vi "Init Shared and Network Variables.vi"(8 "error in (no error)":errorcluster) -> (0 "error out":errorcluster)   [LabVIEW 2024]
uses:
  Type Definitions/FIFO_Health.ctl
  Type Definitions/DIO_Cluster.ctl
  Type Definitions/FPGA_routine_pulsing_typedef.ctl
  Type Definitions/CPU_and_memory.ctl
panel:
  out "current time":timestamp
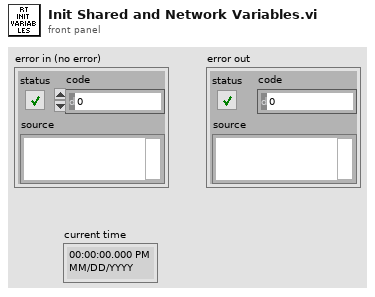
[diagram p1: front panel]
types:
  T1 = typedef "CPU_and_memory.ctl" = cluster{"CPU 1 (%)":dbl, "CPU 2 (%)":dbl, "Free Virtual\nMemory(%)":dbl, "Free Hard drive space (%)":dbl, "Free Physical\n Memory (%)":dbl}
  T2 = typedef "FPGA_routine_pulsing_typedef.ctl" = cluster{"Pulsing":bool, "Pulse duration (uS)":u32, "Pulse Period (uS)":u32}
  T3 = typedef "DIO_Cluster.ctl" = cluster{"DIO0":bool, "DIO1":bool, "DIO2":bool, "DIO3":bool}
  T4 = typedef "FIFO_Health.ctl" = cluster{"Elements in RT FIFO":i32, "Network Stream Full":bool, "RT FIFO Full":bool, "FPGA AI Underflow":bool, "FPGA FIFO Full":bool, "FPGA Loop Timing Off":bool, "timestamp":timestamp, "Stream Size":u32, "Packet Size":u32}
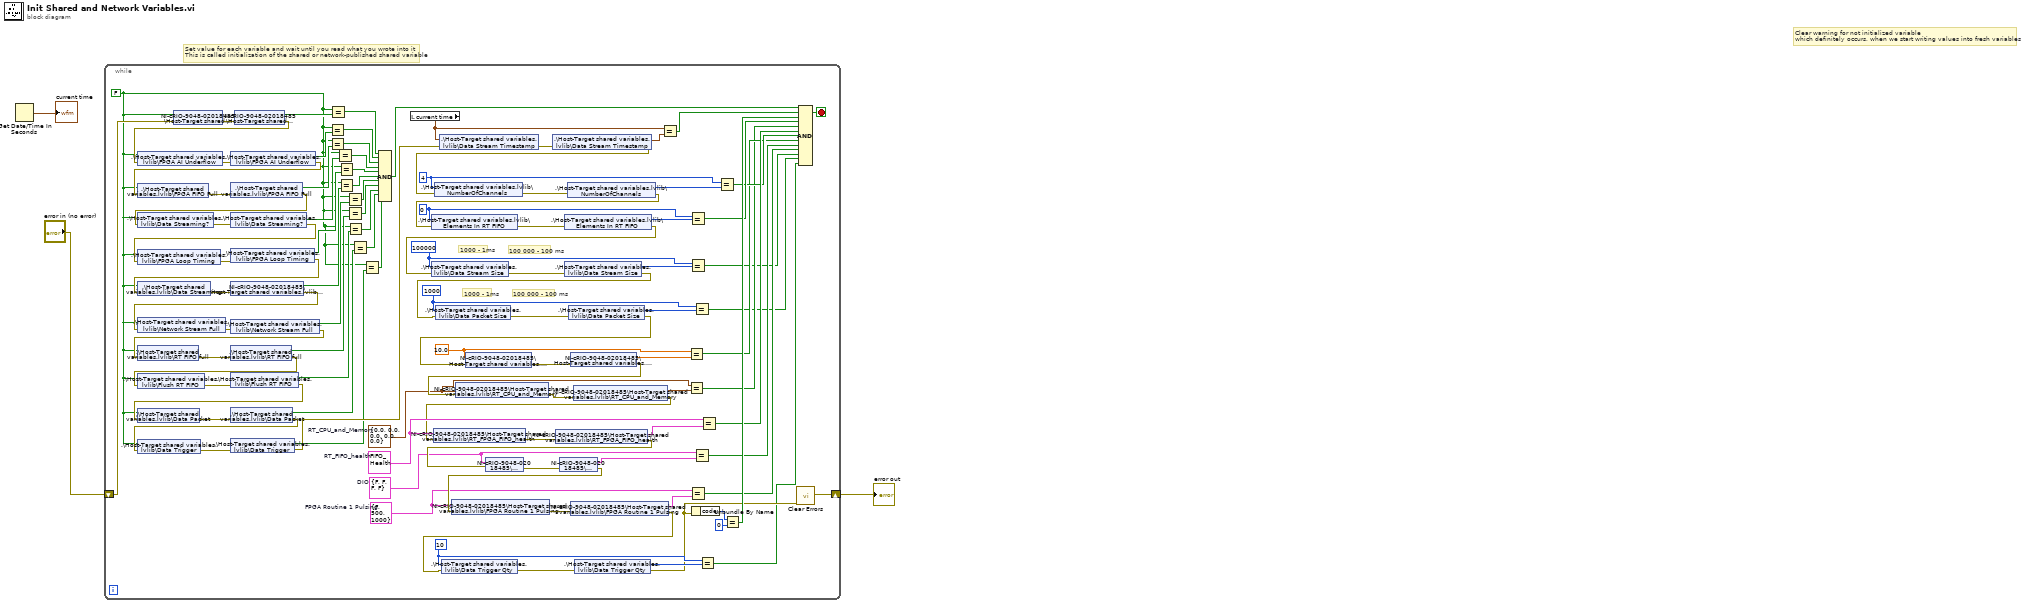
[diagram p0: block diagram]
diagram:
  # "Set value for each variable and wait until you read what you wrote into it\nThis is called initialization of the shared or network-published shared variable"
  # "Clear warning for not initialized variable\nwhich definitely occurs, when we start writing values into fresh variables"
  n1 = Get Date/Time In Seconds() -> (seconds since 1Jan1904=→"current time":timestamp)
  n2 = while {
    shift-right: [w101] -> w2
    shift-left: "error in (no error)" -> [w100]
    stop <- w94 stop-if-true
    w7 = u32 10 ("Elements In RT FIFO AI")
    w19 = u32 1000 ("Elements In RT FIFO AI")
    w24 = u32 100000 ("Elements In RT FIFO AI")
    w45 = T1 {"CPU 1 (%)"=0.0, "CPU 2 (%)"=0.0, "Free Virtual\nMemory(%)"=0.0, "Free Hard drive space (%)"=0.0, "Free Physical\n Memory (%)"=0.0}  # RT_CPU_and_Memory
    w52 = T2 {"Pulsing"=FALSE, "Pulse duration (uS)"=500, "Pulse Period (uS)"=1000}  # FPGA Routine 1 Pulsing
    w56 = T3 {"DIO0"=FALSE, "DIO1"=FALSE, "DIO2"=FALSE, "DIO3"=FALSE}  # DIO
    w61 = 10.0 ("Binning Time")
    w75 = u8 4 ("NumberOfChannels")
    w81 = T4 {"Elements in RT FIFO"=0, "Network Stream Full"=FALSE, "RT FIFO Full"=FALSE, "FPGA AI Underflow"=FALSE, "FPGA FIFO Full"=FALSE, "FPGA Loop Timing Off"=FALSE, "timestamp"=timestamp(0 s since 1904-01-01), "Stream Size"=0, "Packet Size"=0}  # RT_FIFO_health
    w27 = 0 ("Elements In RT FIFO AI")
    w12 = FALSE
    # "100 000 - 100 ms"
    # "1000 - 1ms"
    # "100 000 - 100 ms"
    # "1000 - 1ms"
    n3 = shared-variable "NI-cRIO-9048-02018485\\Host-Target shared variables.lvlib\\Stop RT"(w12, error in=w100) -> (error out=w109:errorcluster)
    n4 = shared-variable "NI-cRIO-9048-02018485\\Host-Target shared variables.lvlib\\Stop RT"(error in=w109) -> (w108:bool, error out=w67:errorcluster)
    n5 = shared-variable ".\\Host-Target shared variables.lvlib\\FPGA AI Underflow"(w12, error in=w67) -> (error out=w43:errorcluster)
    n6 = shared-variable ".\\Host-Target shared variables.lvlib\\FPGA AI Underflow"(error in=w43) -> (w36:bool, error out=w66:errorcluster)
    n7 = shared-variable ".\\Host-Target shared variables.lvlib\\FPGA FIFO Full"(w12, error in=w66) -> (error out=w69:errorcluster)
    n8 = shared-variable ".\\Host-Target shared variables.lvlib\\FPGA FIFO Full"(error in=w69) -> (w35:bool, error out=w68:errorcluster)
    n9 = shared-variable ".\\Host-Target shared variables.lvlib\\Data Streaming?"(w12, error in=w68) -> (error out=w107:errorcluster)
    n10 = shared-variable ".\\Host-Target shared variables.lvlib\\Data Streaming?"(error in=w107) -> (w34:bool, error out=w72:errorcluster)
    n11 = shared-variable ".\\Host-Target shared variables.lvlib\\FPGA Loop Timing"(w12, error in=w72) -> (error out=w73:errorcluster)
    n12 = shared-variable ".\\Host-Target shared variables.lvlib\\FPGA Loop Timing"(error in=w73) -> (w33:bool, error out=w71:errorcluster)
    n13 = shared-variable ".\\Host-Target shared variables.lvlib\\Data Streaming"(w12, error in=w71) -> (error out=w110:errorcluster)
    n14 = shared-variable "NI-cRIO-9048-02018485\\Host-Target shared variables.lvlib\\Data Streaming"(error in=w110) -> (w32:bool, error out=w90:errorcluster)
    n15 = shared-variable ".\\Host-Target shared variables.lvlib\\Network Stream Full"(w12, error in=w90) -> (error out=w92:errorcluster)
    n16 = shared-variable ".\\Host-Target shared variables.lvlib\\Network Stream Full"(error in=w92) -> (w31:bool, error out=w89:errorcluster)
    n17 = shared-variable ".\\Host-Target shared variables.lvlib\\RT FIFO full"(w12, error in=w89) -> (error out=w91:errorcluster)
    n18 = shared-variable ".\\Host-Target shared variables.lvlib\\RT FIFO full"(error in=w91) -> (w30:bool, error out=w41:errorcluster)
    n19 = shared-variable ".\\Host-Target shared variables.lvlib\\Flush RT FIFO"(w12, error in=w41) -> (error out=w42:errorcluster)
    n20 = shared-variable ".\\Host-Target shared variables.lvlib\\Flush RT FIFO"(error in=w42) -> (w40:bool, error out=w37:errorcluster)
    n21 = shared-variable ".\\Host-Target shared variables.lvlib\\Data Packet"(w12, error in=w37) -> (error out=w38:errorcluster)
    n22 = shared-variable ".\\Host-Target shared variables.lvlib\\Data Packet"(error in=w38) -> (w29:bool, error out=w14:errorcluster)
    n23 = shared-variable ".\\Host-Target shared variables.lvlib\\Data Trigger"(w12, error in=w14) -> (error out=w15:errorcluster)
    n24 = shared-variable ".\\Host-Target shared variables.lvlib\\Data Trigger"(error in=w15) -> (w11:bool, error out=w13:errorcluster)
    n25 = Equal?(x=w12, y=w36) -> (x = y?=w105:bool)
    n26 = Equal?(x=w12, y=w35) -> (x = y?=w104:bool)
    n27 = Equal?(x=w12, y=w108) -> (x = y?=w106:bool)
    n28 = Equal?(x=w12, y=w34) -> (x = y?=w88:bool)
    n29 = Equal?(x=w12, y=w33) -> (x = y?=w87:bool)
    n30 = Equal?(x=w12, y=w32) -> (x = y?=w70:bool)
    n31 = Equal?(x=w12, y=w31) -> (x = y?=w64:bool)
    n32 = Equal?(x=w12, y=w30) -> (x = y?=w65:bool)
    n33 = Equal?(x=w12, y=w40) -> (x = y?=w39:bool)
    n34 = Equal?(x=w12, y=w29) -> (x = y?=w28:bool)
    n35 = Equal?(x=w12, y=w11) -> (x = y?=w10:bool)
    n36 = Compound Arithmetic op=AND(w106, w105, w104, w88, w87, w70, w64, w65, w39, w28, w10) -> (w97:bool)
    n37 = local read "current time"() -> (w93:timestamp)
    n38 = shared-variable ".\\Host-Target shared variables.lvlib\\Data Stream Timestamp"(w93, error in=w13) -> (error out=w99:errorcluster)
    n39 = shared-variable ".\\Host-Target shared variables.lvlib\\Data Stream Timestamp"(error in=w99) -> (w98:timestamp, error out=w79:errorcluster)
    n40 = shared-variable ".\\Host-Target shared variables.lvlib\\NumberOfChannels"(w75, error in=w79) -> (error out=w78:errorcluster)
    n41 = shared-variable ".\\Host-Target shared variables.lvlib\\NumberOfChannels"(error in=w78) -> (w76:u8, error out=w77:errorcluster)
    n42 = shared-variable ".\\Host-Target shared variables.lvlib\\Elements In RT FIFO"(w27, error in=w77) -> (error out=w86:errorcluster)
    n43 = shared-variable ".\\Host-Target shared variables.lvlib\\Elements In RT FIFO"(error in=w86) -> (w85:i32, error out=w23:errorcluster)
    n44 = shared-variable ".\\Host-Target shared variables.lvlib\\Data Stream Size"(w24, error in=w23) -> (error out=w26:errorcluster)
    n45 = shared-variable ".\\Host-Target shared variables.lvlib\\Data Stream Size"(error in=w26) -> (w25:u32, error out=w18:errorcluster)
    n46 = shared-variable ".\\Host-Target shared variables.lvlib\\Data Packet Size"(w19, error in=w18) -> (error out=w21:errorcluster)
    n47 = shared-variable ".\\Host-Target shared variables.lvlib\\Data Packet Size"(error in=w21) -> (w20:u32, error out=w17:errorcluster)
    n48 = shared-variable "NI-cRIO-9048-02018485\\Host-Target shared variables.lvlib\\Binning Time"(w61, error in=w17) -> (error out=w63:errorcluster)
    n49 = shared-variable "NI-cRIO-9048-02018485\\Host-Target shared variables.lvlib\\Binning Time"(error in=w63) -> (w62:dbl, error out=w48:errorcluster)
    n50 = shared-variable "NI-cRIO-9048-02018485\\Host-Target shared variables.lvlib\\RT_CPU_and_Memory"(w45, error in=w48) -> (error out=w49:errorcluster)
    n51 = shared-variable "NI-cRIO-9048-02018485\\Host-Target shared variables.lvlib\\RT_CPU_and_Memory"(error in=w49) -> (w46:T1, error out=w47:errorcluster)
    n52 = shared-variable "NI-cRIO-9048-02018485\\Host-Target shared variables.lvlib\\RT_FPGA_FIFO_health"(w81, error in=w47) -> (error out=w83:errorcluster)
    n53 = shared-variable "NI-cRIO-9048-02018485\\Host-Target shared variables.lvlib\\RT_FPGA_FIFO_health"(error in=w83) -> (w82:T4, error out=w59:errorcluster)
    n54 = shared-variable "NI-cRIO-9048-02018485\\Host-Target shared variables.lvlib\\DIO"(w56, error in=w59) -> (error out=w58:errorcluster)
    n55 = shared-variable "NI-cRIO-9048-02018485\\Host-Target shared variables.lvlib\\DIO"(error in=w58) -> (w57:T3, error out=w54:errorcluster)
    n56 = shared-variable "NI-cRIO-9048-02018485\\Host-Target shared variables.lvlib\\FPGA Routine 1 Pulsing"(w52, error in=w54) -> (error out=w53:errorcluster)
    n57 = shared-variable "NI-cRIO-9048-02018485\\Host-Target shared variables.lvlib\\FPGA Routine 1 Pulsing"(error in=w53) -> (w51:T2, error out=w6:errorcluster)
    n58 = shared-variable ".\\Host-Target shared variables.lvlib\\Data Trigger Qty"(w7, error in=w6) -> (error out=w9:errorcluster)
    n59 = shared-variable ".\\Host-Target shared variables.lvlib\\Data Trigger Qty"(error in=w9) -> (w8:u32, error out=w5:errorcluster)
    n60 = Equal?(x=w93, y=w98) -> (x = y?=w96:bool)
    n61 = Equal?(x=w61, y=w62) -> (x = y?=w60:bool)
    n62 = Equal?(x=w45, y=w46) -> (x = y?=w44:bool)
    n63 = Equal?(x=w27, y=w85) -> (x = y?=w84:bool)
    n64 = Equal?(x=w24, y=w25) -> (x = y?=w22:bool)
    n65 = Equal?(x=w52, y=w51) -> (x = y?=w50:bool)
    n66 = Unbundle By Name(w5) -> ("code"=w103:i32)
    n67 = Equal?(x=w19, y=w20) -> (x = y?=w16:bool)
    n68 = Equal?(x=w56, y=w57) -> (x = y?=w55:bool)
    n69 = Equal?(x=w7, y=w8) -> (x = y?=w4:bool)
    n70 = Equal?(x=w81, y=w82) -> (x = y?=w80:bool)
    n71 = Equal?(x=w75, y=w76) -> (x = y?=w74:bool)
    n72 = Equal?(x=w103, y=0) -> (x = y?=w95:bool)
    n73 = call <vilib>:"Clear Errors.vi"("error in (no error)"=w5) -> ("error out"=w101:errorcluster)  [unwired: 5 in, 1 out]
    n74 = Compound Arithmetic op=AND(w97, w96, w95, w84, w44, w80, w74, w60, w55, w50, w22, w16, w4) -> (w94:bool)
  }
  "error out" <- w2
